vi "Get All Impulses.vi"(8 "error in (no error)":errorcluster, 11 "Impulse Manager in":refnum<class "Impulse Manager.lvclass">) -> (0 "error out":errorcluster, 2 "Data out":cluster{"Impulses out":dbl[][]}[](array[cluster]), 3 "Impulse Manager out":refnum<class "Impulse Manager.lvclass">)   [LabVIEW 2013, in "Impulse Manager.lvclass"]
uses:
  Impulse Manager.lvclass
  Impulse Manager.lvclass/Impulse Manager.ctl
  Impulse Data/Impulse Data.lvclass
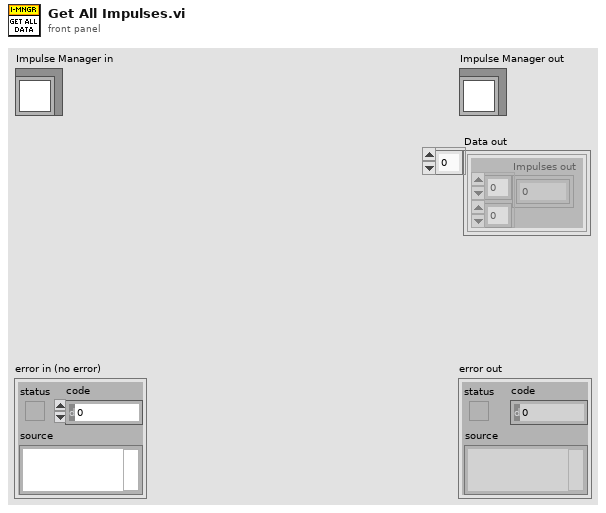
[diagram p1: front panel]
types:
  T1 = typedef "Impulse Data.lvclass/Instance handle.ctl" = refnum<data-value>
  T2 = typedef "core.lvlib/TD_Impulse Parameter.ctl" = cluster{"Color":u32, "Visible":bool, "Channel":u16, "Invert":bool, "Desaccade":bool, "Offset":dbl, "Gain":dbl}[]
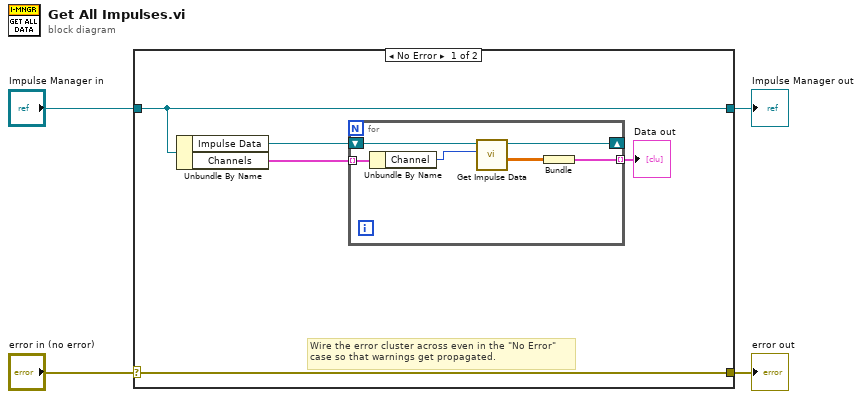
[diagram p0: block diagram]
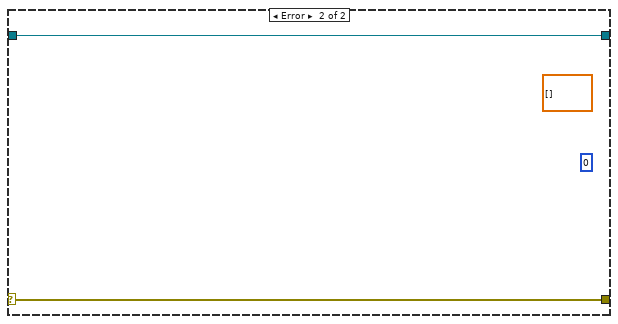
[diagram p2: hidden frame]
diagram:
  n1 = case shown="No Error" "error in (no error)" {
    selector: "error in (no error)" -> [w9 w17]
    tunnel: [w9 w17] -> w3
    tunnel: [w8 w16] -> w1
    tunnel: "Impulse Manager in" -> [w8 w16]
    frame No Error {
      # "Wire the error cluster across even in the \"No Error\"\ncase so that warnings get propagated."
      n2 = Unbundle By Name(w8) -> ("Impulse Data"=w6:T1, "Channels"=w7:T2)
      n3 = for {
        tunnel: w7 -> [w13] mode=indexing
        shift-right: [w14] -> _
        shift-left: w6 -> [w15]
        tunnel: [w10] -> w5 mode=indexing
        n4 = Unbundle By Name(w13) -> ("Channel"=w12:u16)
        n5 = call "Get Impulse Data.vi"("Channel"=w12, "Reference in"=w15) -> ("Impulses out"=w11:dbl[][], "Reference out"=w14:T1)  [unwired: 8 in]
        n6 = Bundle("Impulses out"=w11) -> (w10:cluster{"Impulses out":dbl[][]})  [unwired: 1 in]
      }
      "Data out" <- w5
    }
    frame Error {
      (unwired) 0
      (unwired) dbl[][] [] ("Impulses out")
    }
  }
  "error out" <- w3
  "Impulse Manager out" <- w1
